vi "crh_xcopyAll.vi"(11 "folder":string="QAMT02\\CRH3605_95TH248") -> ()   [LabVIEW 2012]
panel:
  out "concatenated string":string
  out "OK 2":bool
  out "concatenated string 2":string
  out "folder 2":string
  out "OK":bool
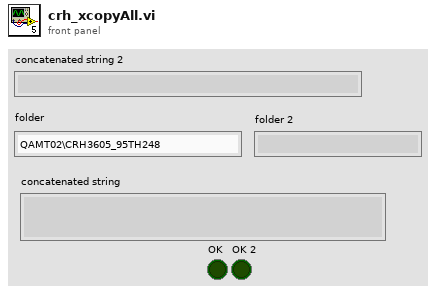
[diagram p1: front panel]
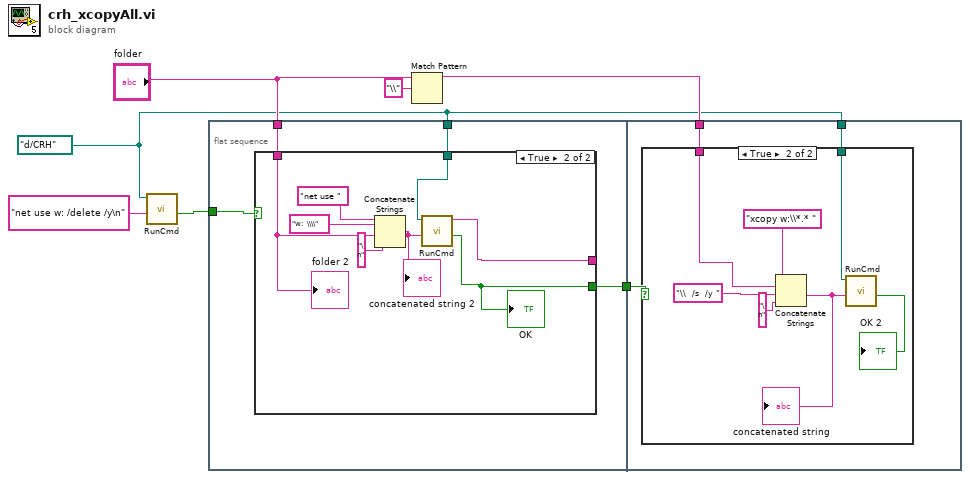
[diagram p0: block diagram]
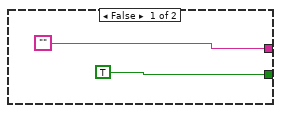
[diagram p2: hidden frame]
diagram:
  w1 = path "d:/CRH" ("working directory")
  n1 = call "RunCmd.vi"("Cmd String"="net use w: /delete /y\n" ("string"), "working directory"=w1) -> ("OK"=w4:bool)  [unwired: 8 in, 1 out]
  n2 = flat-sequence {
    tunnel: "folder" -> [w10]
    tunnel: w1 -> [w9]
    tunnel: w4 -> [w8]
    tunnel: [w11] -> w3
    tunnel: w3 -> [w22]
    tunnel: w2 -> [w24]
    tunnel: w1 -> [w23]
    frame #0 {
      n3 = case shown="True" w8 {
        tunnel: [TRUE w15] -> w11
        tunnel: ["" w16] -> _
        tunnel: w10 -> [_ w18]
        tunnel: w9 -> [_ w17]
        frame False {
        }
        frame True {
          n4 = Concatenate Strings("net use " ("string"), "w:  \\\\" ("string"), w18, "\n" ("string")) -> (w21:string)
          "concatenated string 2" <- w21
          n5 = call "RunCmd.vi"("Cmd String"=w21, "working directory"=w17) -> ("OK"=w15:bool, "Output"=w16:string)  [unwired: 8 in]
          "OK" <- w15
          "folder 2" <- w18
        }
      }
    }
    frame #1 {
      n6 = case shown="True" w22 {
        tunnel: w24 -> [_ w31]
        tunnel: w23 -> [_ w28]
        frame False {
        }
        frame True {
          n7 = Concatenate Strings("xcopy w:\\*.* " ("string"), w31, "\\  /s  /y " ("string"), "\n" ("string")) -> (w27:string)
          "concatenated string" <- w27
          n8 = call "RunCmd.vi"("Cmd String"=w27, "working directory"=w28) -> ("OK"=→"OK 2":bool)  [unwired: 8 in, 1 out]
        }
      }
    }
  }
  n9 = Match Pattern(string="folder", regular expression="\\") -> (before substring=w2:string)  [unwired: 1 in, 3 out]
